vi "WalkOnAssertions.vi"(6 "Stop on 1st fail":bool, 7 "Banana":refnum<class "Banana.lvclass">, 8 "error in (no error)":errorcluster, 11 "Leaf.Assertion":refnum<class "Leaf.Assertion.lvclass">) -> (0 "error out":errorcluster, 3 "Leaf.Assertion":refnum<class "Leaf.Assertion.lvclass">)   [LabVIEW 2021, in "Bananas.lvlib" / "Platano.lvclass"]
uses:
  Platano.lvclass
  Banana/Banana.lvclass
  Banana/Banana.lvclass/Banana.ctl
  BananaPeel/BananaPeel.lvclass
  Leaf.Assertion/Leaf.Assertion.lvclass
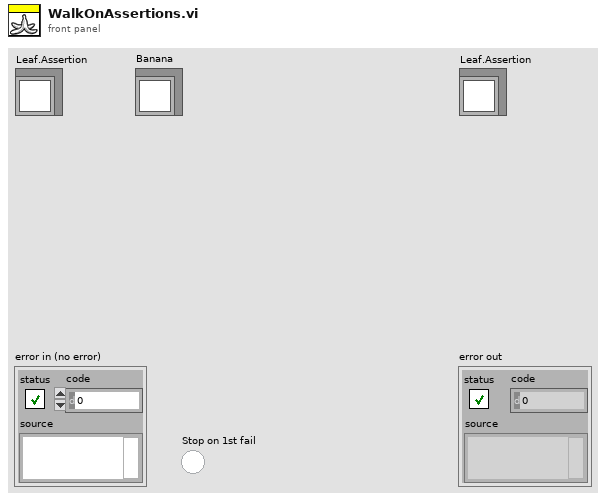
[diagram p1: front panel]
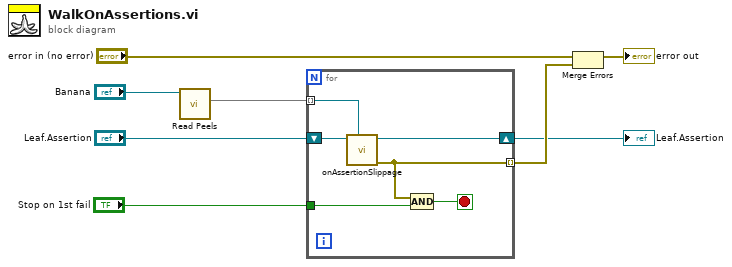
[diagram p0: block diagram]
diagram:
  n1 = call "Read Peels.vi"("Banana in"="Banana") -> ("Peels"=w1:set{refnum<class "BananaPeel.lvclass">})  [unwired: 8 in, 2 out]
  n2 = for {
    tunnel: [w13] -> w8 mode=indexing
    shift-right: [w9] -> w5
    shift-left: "Leaf.Assertion" -> [w10]
    tunnel: w1 -> [w14] mode=indexing
    tunnel: "Stop on 1st fail" -> [w12]
    stop <- w11 stop-if-true
    n3 = call-dynamic "onAssertionSlippage.vi"("BananaPeel in"=w14, "Leaf.Assertion"=w10) -> ("error out"=w13:errorcluster, "Leaf.Assertion"=w9:refnum<class "Leaf.Assertion.lvclass">)  [unwired: 8 in]
    n4 = Compound Arithmetic op=AND(w13, w12) -> (w11:bool)
  }
  "Leaf.Assertion" <- w5
  n5 = Merge Errors("error in (no error)", w8) -> (→"error out":errorcluster)
